vi "KickValueTest.vi"(8 "error in (no error)":errorcluster, 9 "grSIM replacement":T6, 10 "KickValueTest":T3={"ForceValue"={"delta_kick"=0.0, "kick_min"=1.0, "kick_max"=0.0}, "BallValue"={"delta_ball"=0.0, "v_min_ball"=1.0, "v_max_ball"=0.0}, "Samples"=0.0, "Start"=FALSE, "id"=0, "RobotStopKick"=FALSE}, 11 "Game in":refnum<class "Game.lvclass">) -> (0 "error out":errorcluster, 1 "KickValueState":T1 {"Progress" scale=0.0..100.0}, 2 "grSIM replacement out":T6, 3 "Game out":refnum<class "Game.lvclass">, 4 "replaceBall":bool, 5 "TestTeam":refnum<class "Ally.lvclass">, 6 "KickValue":dbl[][](array[numeric]), 7 "replaceRobots":bool)   [LabVIEW 2021, in "Game.lvclass"]
uses:
  Game.lvclass
  Controls/grSimReplacement.ctl
  Communication_class/Paths/grSim Packet Command UDP Test Folder/grSim/grSim RobotReplacement.ctl
  Communication_class/Paths/grSim Packet Command UDP Test Folder/grSim/grSim_BallReplacement.ctl
  Ally_class/Ally.lvclass
  D:/RoboIme/horie/SSL_AI/Team_class/Team.lvclass
  KickValuetest.ctl
  KickValue.ctl
  BallValue.ctl
  Kickvaluestate.ctl
  KickForceTest/Controls/KickForceEnum.ctl
  Game.lvclass/Game.ctl
  Team_class/Team.lvclass/Team.ctl
  Ball_class/Ball.lvclass/Ball.ctl
  Object_class/Object.lvclass/Object.ctl
  Robot_class/Robot.lvclass/Robot.ctl
  Events_class/Events.lvclass/Events.ctl
  RobotFeedback/RobotFeedback.lvclass/RobotFeedback.ctl
  <vilib>/Analysis/_algsub.llb/Real Vector Norm.vi
  Object_class/Read position(x,y).vi
  Events_class/Read kick.vi
  RobotFeedback/Read dribblerContactToBall.vi
  Robot_class/Write kick_x.vi
  Robot_class/Write v_tang.vi
  Robot_class/Write dribble.vi
  Read TestTeam.vi
  Read Utilities.lvclass.vi
  Read AllyRef.vi
  Read BallRef.vi
  Read FieldRef.vi
  Read EventsRef.vi
  Read RobotsFeedback.vi
  Ball_class/Read v_x.vi
  Ball_class/Read v_y.vi
  Object_class/Read x.vi
  Object_class/Read y.vi
  Team_class/Read RobotRef.vi
  Team_class/Write RobotRef.vi
  Ball_class/Ball.lvclass
  D:/RoboIme/horie/SSL_AI/Object_class/Object.lvclass
  Robot_class/Robot.lvclass
  Utilities_class/Utilities.lvclass
  Field_class/Field.lvclass
  Events_class/Events.lvclass
  RobotFeedback/RobotFeedback.lvclass
  <vilib>/Analysis/NI_AALPro.lvlib
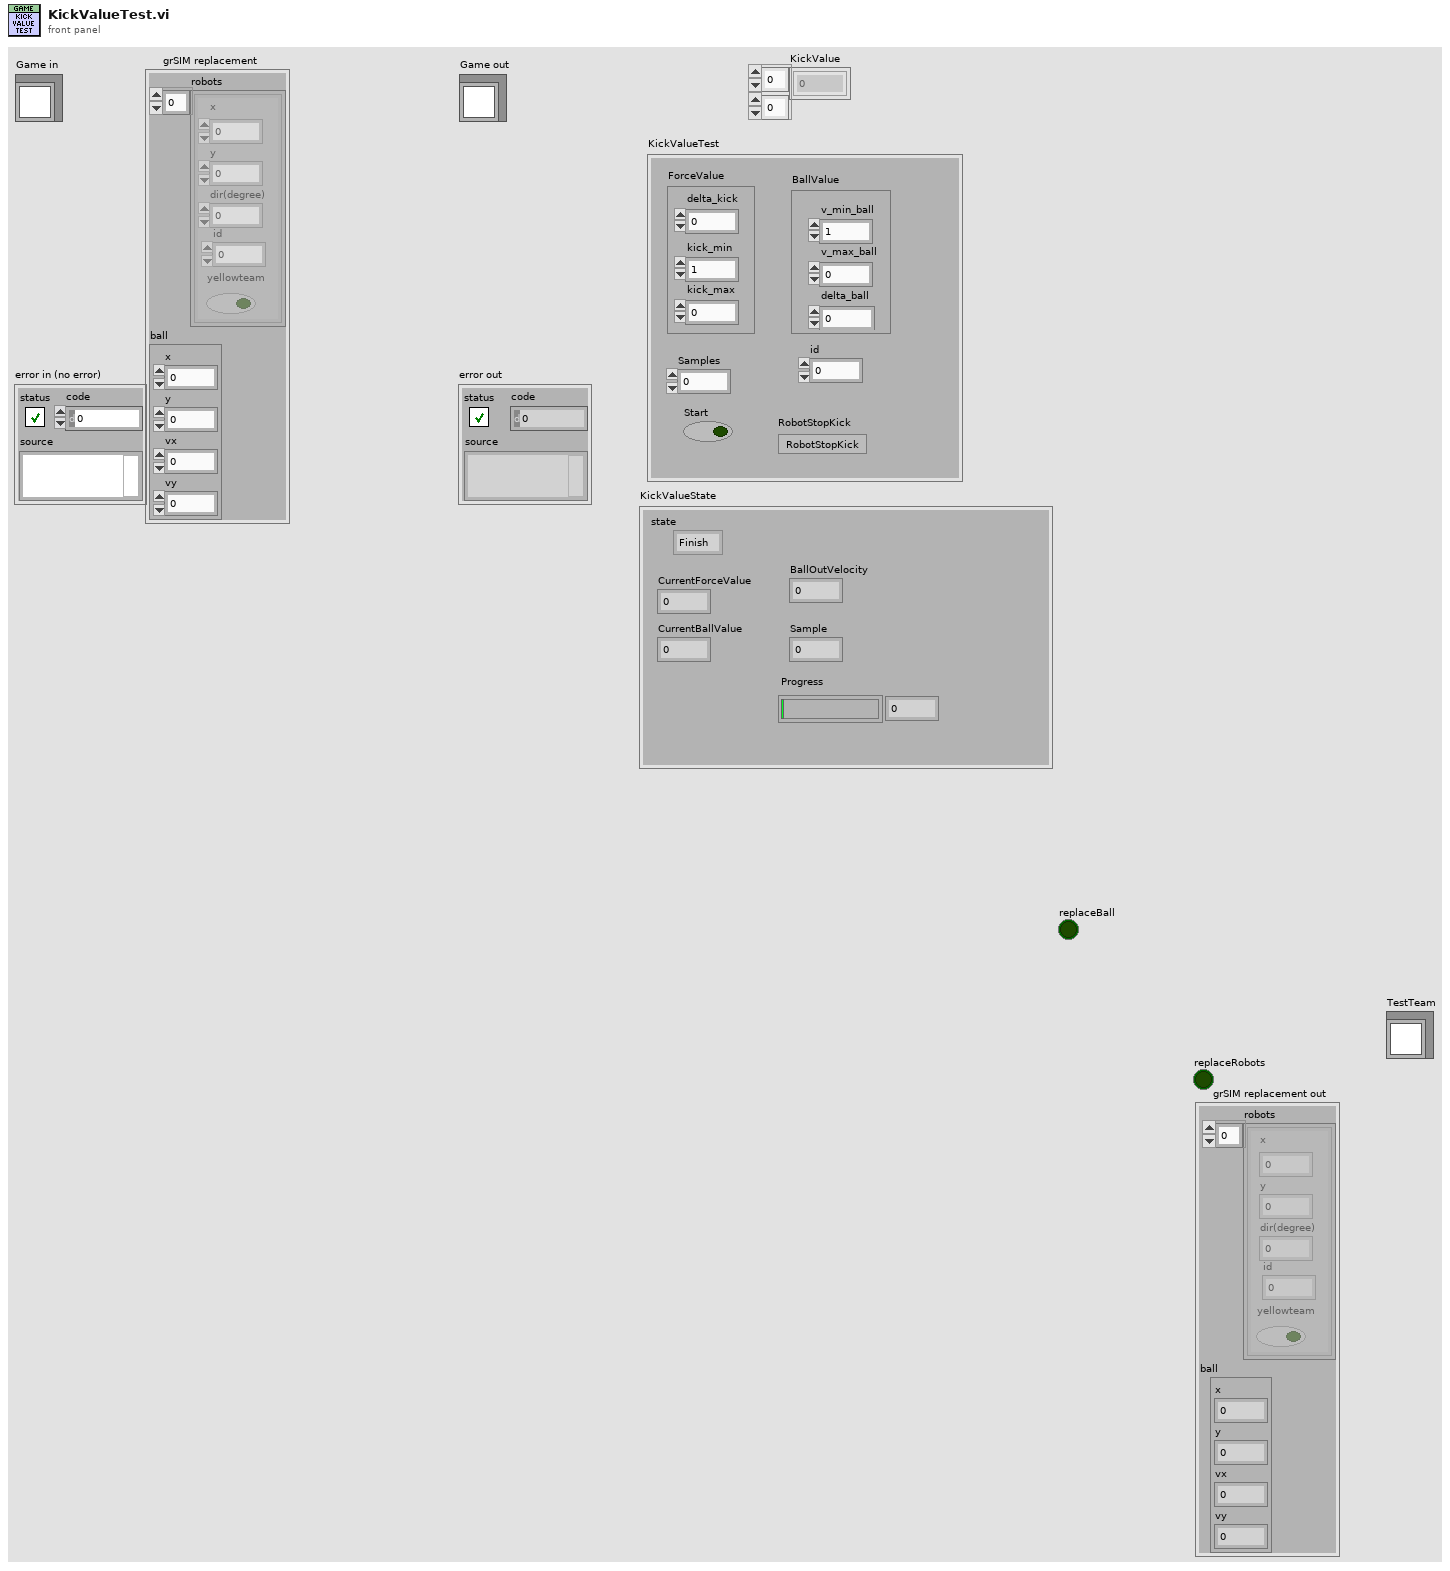
[diagram p1: front panel]
types:
  T1 = typedef "Game.lvclass/Kickvaluestate.ctl" = cluster{"state":T2, "CurrentForceValue":dbl, "CurrentBallValue":dbl, "BallOutVelocity":dbl, "Sample":dbl, "Progress":dbl}
  T2 = typedef "Game.lvclass/KickForceEnum.ctl" = enum16{"Finish", "Velball", "GoToNextKickForce", "WaitBall", "KickBall", "ReplaceBall"}
  T3 = typedef "KickValuetest.ctl" = cluster{"ForceValue":T4, "BallValue":T5, "Samples":dbl, "Start":bool, "id":i32, "RobotStopKick":bool}
  T4 = typedef "Game.lvclass/KickValue.ctl" = cluster{"delta_kick":dbl, "kick_min":dbl, "kick_max":dbl}
  T5 = typedef "Game.lvclass/BallValue.ctl" = cluster{"delta_ball":dbl, "v_min_ball":dbl, "v_max_ball":dbl}
  T6 = typedef "grSimReplacement.ctl" = cluster{"robots":T7[], "ball":T8}
  T7 = typedef "grSim RobotReplacement.ctl" = cluster{"x":dbl, "y":dbl, "dir(degree)":dbl, "yellowteam":bool, "id":u32}
  T8 = typedef "grSim_BallReplacement.ctl" = cluster{"x":dbl, "y":dbl, "vx":dbl, "vy":dbl}
  T9 = typedef "Kickmeanvalues.ctl" = dbl[][]
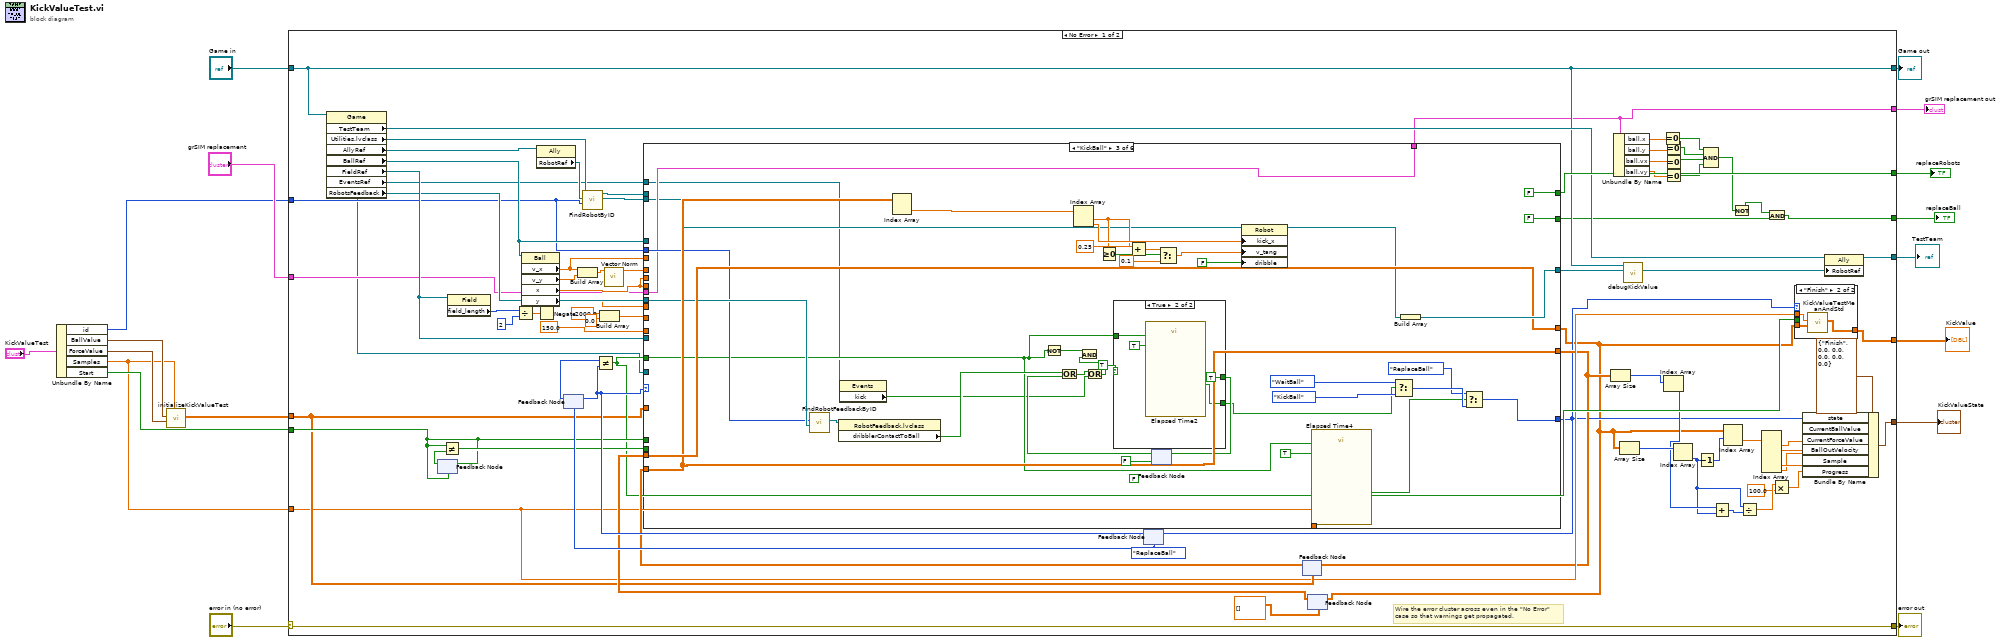
[diagram p0: block diagram]
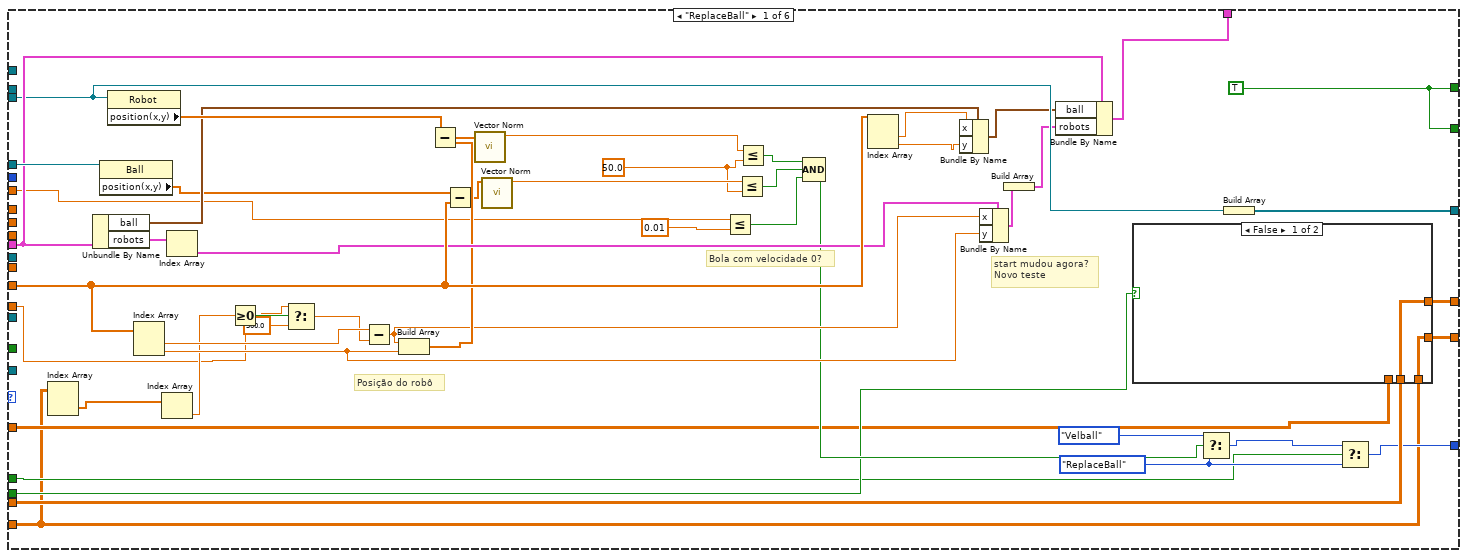
[diagram p3: hidden frame]
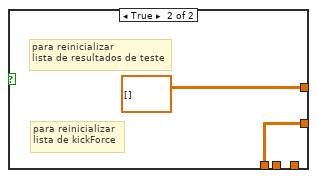
[diagram p4: hidden frame]
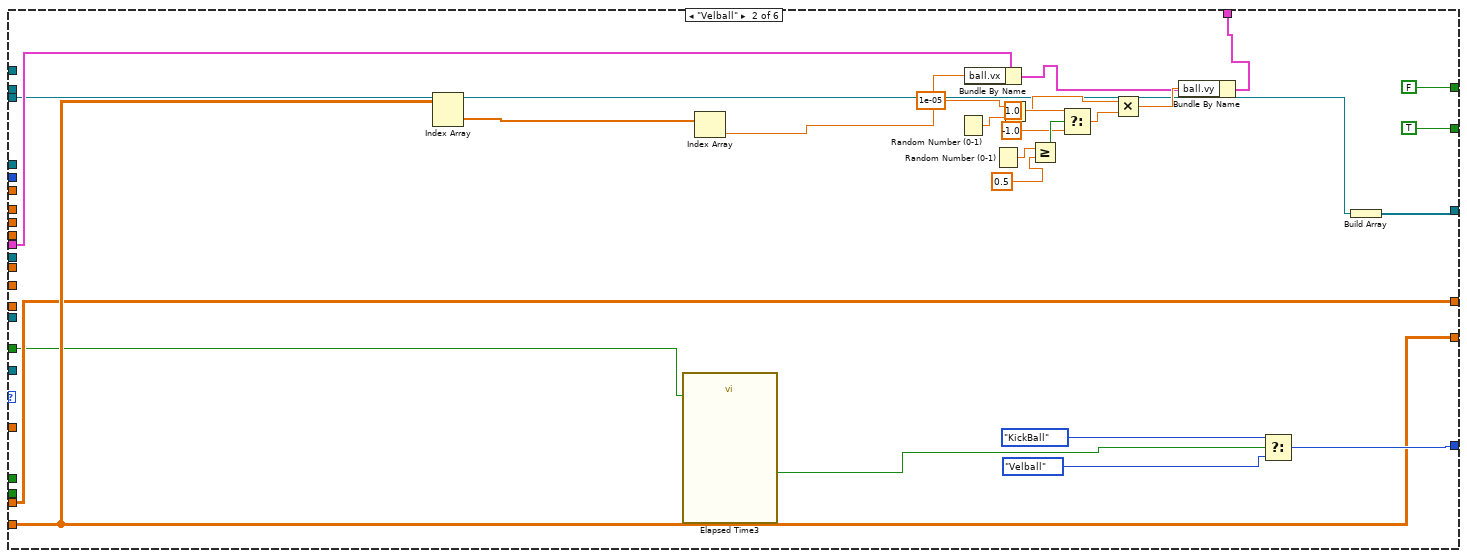
[diagram p5: hidden frame]
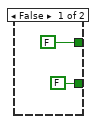
[diagram p6: hidden frame]
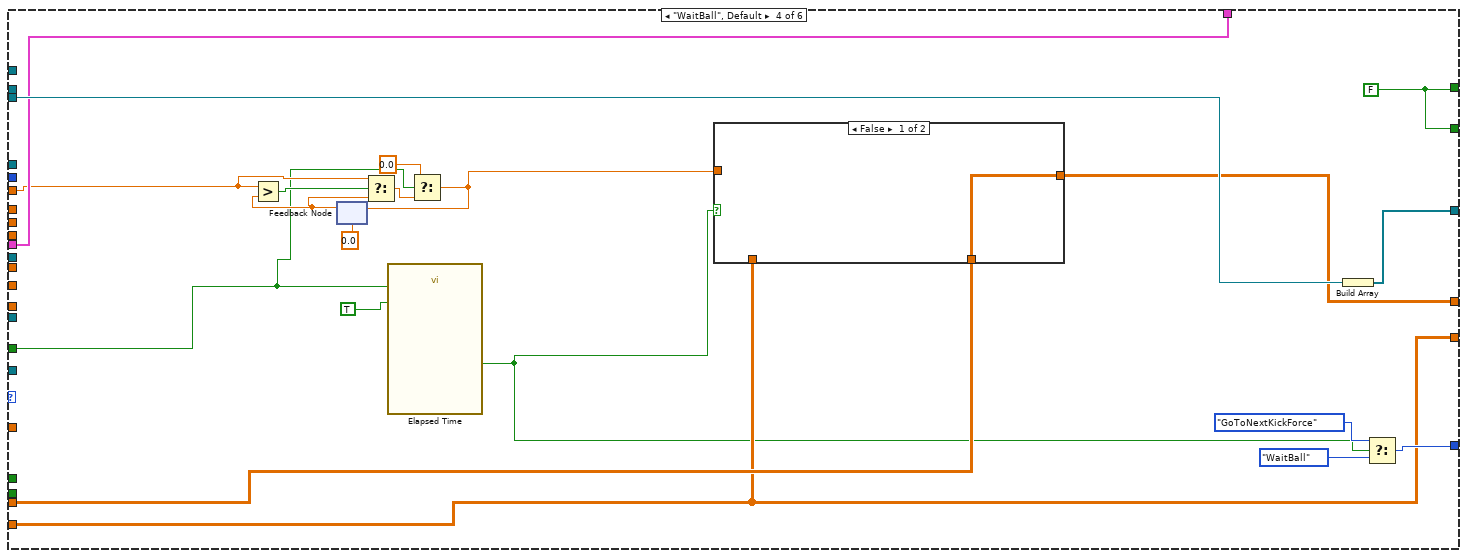
[diagram p7: hidden frame]
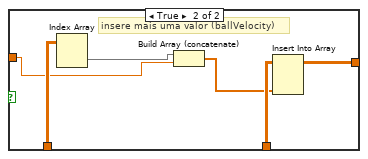
[diagram p8: hidden frame]
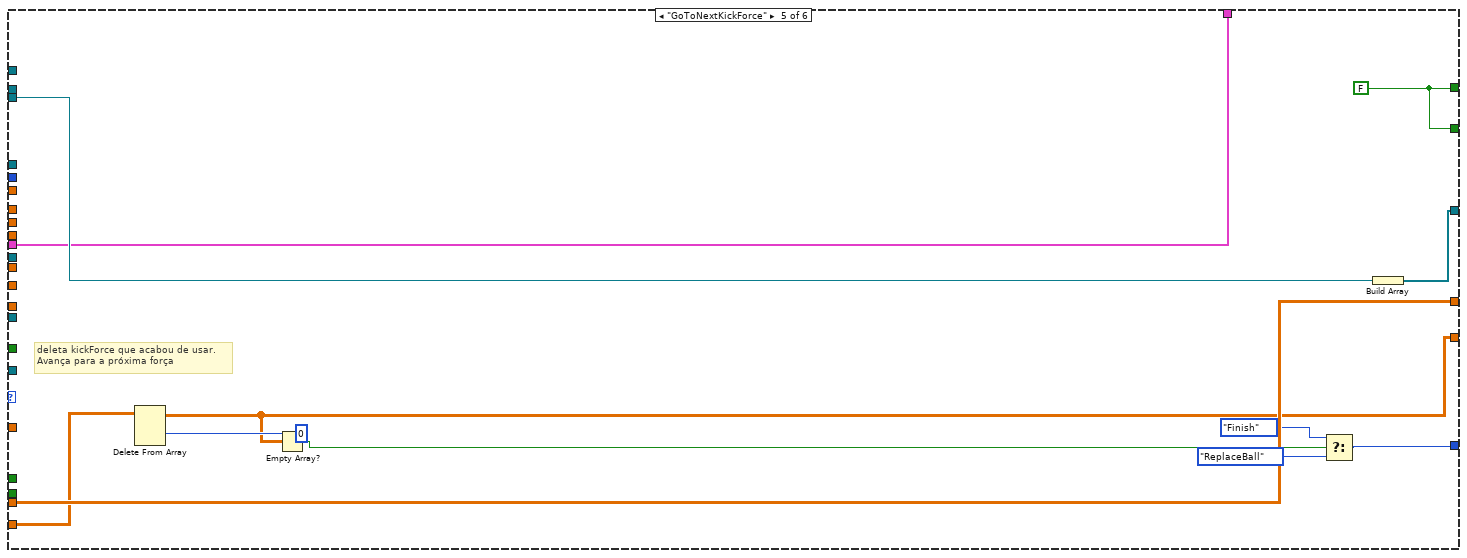
[diagram p9: hidden frame]
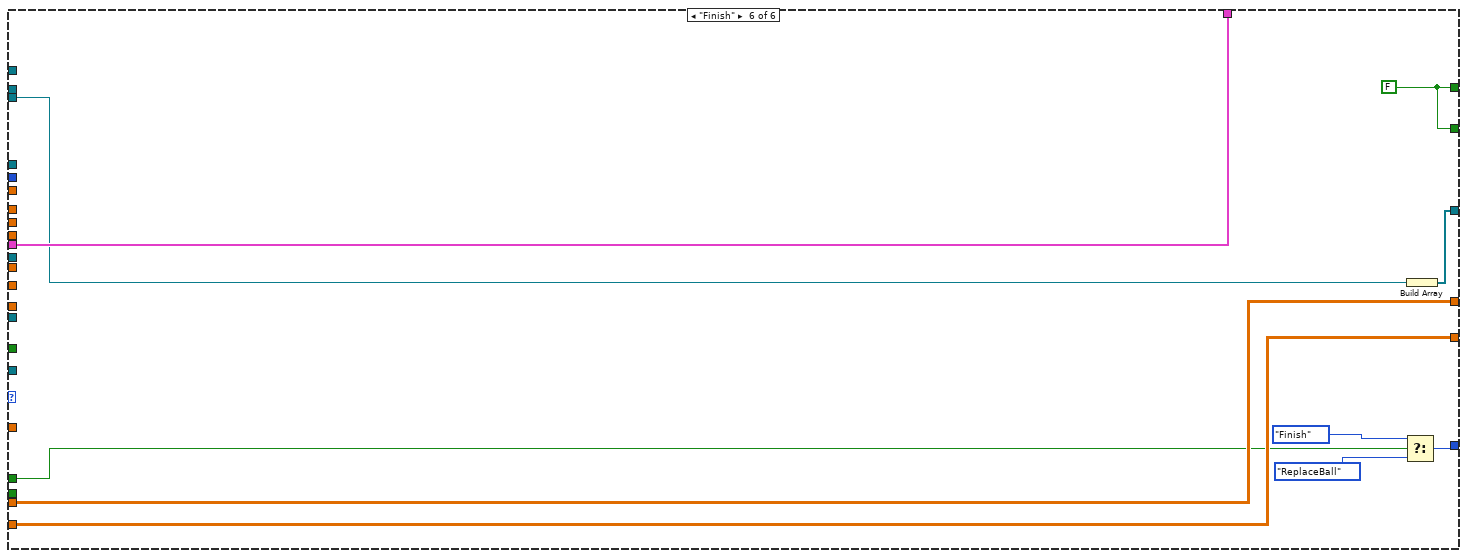
[diagram p10: hidden frame]
diagram:
  n1 = Unbundle By Name("KickValueTest") -> ("id"=w10:i32, "BallValue"=w11:T5, "ForceValue"=w12:T4, "Samples"=w7:dbl, "Start"=w9:bool)
  n2 = call "initializeKickValueTest.vi"("samples"=w7, "ForceValue"=w12, "BallValue"=w11) -> ("kickForceList"=w8:dbl[][])  [unwired: 6 in, 2 out]
  n3 = case shown="No Error" "error in (no error)" {
    selector: "error in (no error)" -> [w94 w272]
    tunnel: [w94 w272] -> w17
    tunnel: [w55 w271] -> w15
    tunnel: "Game in" -> [w55 w271]
    tunnel: w10 -> [w52 _]
    tunnel: w9 -> [w74 _]
    tunnel: "grSIM replacement" -> [w40 _]
    tunnel: w8 -> [w59 _]
    tunnel: w7 -> [w23 _]
    tunnel: [w70 _] -> w6
    tunnel: [w35 _] -> w5
    tunnel: [w69 _] -> w4
    tunnel: [w58 _] -> w3
    tunnel: [w67 _] -> w2
    tunnel: [w37 _] -> w1
    frame No Error {
      w77 = KickForceEnum."ReplaceBall" ("kickForceEnum")
      # "Wire the error cluster across even in the \"No Error\"\ncase so that warnings get propagated."
      n4 = property class="Game"(reference=w55) -> ("TestTeam"=w68:refnum<class "Ally.lvclass">, "Utilities.lvclass"=w91:refnum<class "Utilities.lvclass">, "AllyRef"=w93:refnum<class "Ally.lvclass">, "BallRef"=w86:refnum<class "Ball.lvclass">, "FieldRef"=w82:refnum<class "Field.lvclass">, "EventsRef"=w19:refnum<class "Events.lvclass">, "RobotsFeedback"=w53:refnum<class "RobotFeedback.lvclass">[])  [unwired: 1 in, 2 out]
      n5 = feedback #1(w74) -> (w76:bool)
      n6 = feedback-in #1(w74) -> ()
      n7 = Not Equal?(x=w74, y=w76) -> (x != y?=w75:bool)
      n8 = property class="Field"(reference=w82) -> ("field_length"=w85:i32)  [unwired: 1 in, 2 out]
      n9 = Divide(x=w85, y=2) -> (x/y=w83:dbl)
      n10 = property class="Ball"(reference=w86) -> ("v_x"=w54:dbl, "v_y"=w88:dbl, "x"=w42:dbl, "y"=w41:dbl)  [unwired: 1 in, 2 out]
      n11 = property class="Ally"(reference=w93) -> ("RobotRef"=w92:refnum<class "Robot.lvclass">[])  [unwired: 1 in, 2 out]
      n12 = Negate(x=w83) -> ()  [unwired: 1 out]
      n13 = feedback #2(w77) -> (w79:T2)
      n14 = Build Array(w54, w88) -> (w87:dbl[])
      n15 = call "FindRobotByID.vi"("id"=w52, "RobotRef"=w92, "Utilities in"=w91) -> ("Robot"=w89:refnum<class "Robot.lvclass">, "Utilities out"=w90:refnum<class "Utilities.lvclass">)  [unwired: 5 in, 2 out]
      n16 = Build Array(-2000.0 ("element"), 0.0 ("element")) -> (w81:dbl[])
      n17 = call-poly <vilib>:"Vector Norm.vi"("Input Vector"=w87) -> ("norm"=w36:dbl)  [unwired: 9 in, 1 out]
      n18 = feedback #3(w77) -> (w78:T2)
      n19 = feedback-in #2(w78) -> ()
      n20 = Not Equal?(x=w79, y=w78) -> (x != y?=w60:bool)
      n21 = feedback #4(w59) -> (w73:dbl[][])
      n22 = feedback #5(dbl[][] []) -> (w71:dbl[][])
      n23 = case shown="\"KickBall\"" w78 {
        tunnel: [w141 w173 w215 w240 w257 w266] -> w57
        tunnel: [w110 FALSE ("replaceRobots") FALSE ("replaceRobots") w232 w249 w261] -> w70
        tunnel: w89 -> [w142 w157 w188 w241 w256 w267]
        tunnel: w86 -> [w146 _ _ _ _ _]
        tunnel: w40 -> [w145 w170 w189 w235 w255 w270]
        tunnel: [w144 w156 w189 w235 w255 w270] -> w35
        tunnel: w81 -> [w143 _ _ _ _ _]
        tunnel: 150.0 ("y") -> [w99 _ _ _ _ _]
        tunnel: [w106 w174 w185 w237 w251 w264] -> w21
        tunnel: w54 -> [w115 _ _ w228 _ _]
        tunnel: w71 -> [w116 w153 w213 w239 w260 w269]
        tunnel: [w140 w153 w213 w238 w260 w269] -> w20
        tunnel: w73 -> [w104 w169 w211 w236 w259 w268]
        tunnel: w82 -> [_ _ _ _ _ _]
        tunnel: [w118 w169 w211 w236 w250 w268] -> w22
        tunnel: w60 -> [_ w151 w182 w225 _ _]
        tunnel: w74 -> [w105 _ _ _ _ w265]
        tunnel: w59 -> [w111 _ _ _ _ _]
        tunnel: w90 -> [_ _ _ _ _ _]
        tunnel: w75 -> [w117 _ _ _ _ _]
        tunnel: w23 -> [_ _ _ _ _ _]
        tunnel: [w110 TRUE ("replaceRobots") FALSE ("replaceRobots") w232 w249 w261] -> w39
        tunnel: w19 -> [_ _ _ _ _ _]
        tunnel: w53 -> [_ _ w199 _ _ _]
        tunnel: w52 -> [_ _ w198 _ _ _]
        tunnel: w42 -> [_ _ _ _ _ _]
        tunnel: w42 -> [_ _ _ _ _ _]
        tunnel: w41 -> [_ _ _ _ _ _]
        tunnel: w36 -> [_ _ _ _ _ _]
        tunnel: w19 -> [_ _ w181 _ _ _]
        frame "ReplaceBall" {
          w107 = KickForceEnum."ReplaceBall" ("kickForceEnum")
          w120 = 50.0 ("y")
          w110 = TRUE ("replaceRobots")
          # "Bola com velocidade 0?"
          # "start mudou agora?\nNovo teste"
          # "Posição do robô"
          n24 = Index Array(array=w104) -> (element=w103:dbl[])  [unwired: 2 in]
          n25 = Unbundle By Name(w145) -> ("ball"=w135:T8, "robots"=w139:T7[])
          n26 = property class="Ball"(reference=w146) -> ("position(x,y)"=w123:dbl[])  [unwired: 1 in, 2 out]
          n27 = property class="Robot"(reference=w142) -> ("position(x,y)"=w138:dbl[])  [unwired: 1 in, 2 out]
          n28 = Index Array(array=w143) -> (element #1=w129:dbl, element #2=w126:dbl)  [unwired: 2 in]
          n29 = Index Array(array=w103) -> (element=w100:dbl)  [unwired: 1 in]
          n30 = Index Array(array=w139) -> (element=w133:T7)  [unwired: 1 in]
          n31 = Greater Or Equal To 0?(x=w100) -> (x >= 0?=w102:bool)
          n32 = Select(t=w99, s=w102, f=300.0) -> (s? t:f=w101:dbl)
          n33 = Subtract(x=w129, y=w101) -> (x-y=w127:dbl)
          n34 = Build Array(w127, w126) -> (w128:dbl[])
          n35 = Subtract(x=w138, y=w128) -> (x-y=w137:dbl[])
          n36 = Subtract(x=w123, y=w143) -> (x-y=w122:dbl[])
          n37 = call-poly <vilib>:"Vector Norm.vi"("Input Vector"=w137) -> ("norm"=w136:dbl)  [unwired: 9 in, 1 out]
          n38 = call-poly <vilib>:"Vector Norm.vi"("Input Vector"=w122) -> ("norm"=w121:dbl)  [unwired: 9 in, 1 out]
          n39 = Less Or Equal?(x=w115, y=0.01) -> (x <= y?=w113:bool)
          n40 = Less Or Equal?(x=w121, y=w120) -> (x <= y?=w119:bool)
          n41 = Less Or Equal?(x=w136, y=w120) -> (x <= y?=w125:bool)
          n42 = Compound Arithmetic op=AND(w125, w119, w113) -> (w124:bool)
          n43 = Index Array(array=w143) -> (element #1=w132:dbl, element #2=w109:dbl)  [unwired: 2 in]
          n44 = Bundle By Name(cluster=w135, "x"=w132, "y"=w109) -> (w134:T8)
          n45 = Bundle By Name(cluster=w133, "x"=w127, "y"=w126) -> (w131:T7)
          n46 = Build Array(w131) -> (w130:T7[])
          n47 = Bundle By Name(cluster=w145, "ball"=w134, "robots"=w130) -> (w144:T6)
          n48 = case shown="False" w117 {
            tunnel: [w148 dbl[][] []] -> w140
            tunnel: [w147 w149] -> w118
            tunnel: w111 -> [_ w149]
            tunnel: w116 -> [w148 _]
            tunnel: w104 -> [w147 _]
            frame False {
            }
            frame True {
              # "para reinicializar\nlista de resultados de teste"
              # "para reinicializar\nlista de kickForce"
            }
          }
          n49 = Select(t=KickForceEnum."Velball" ("kickForceEnum"), s=w124, f=w107) -> (s? t:f=w108:T2)
          n50 = Build Array(w142) -> (w141:refnum<class "Robot.lvclass">[])
          n51 = Select(t=w108, s=w105, f=w107) -> (s? t:f=w106:T2)
        }
        frame "Velball" {
          n52 = Index Array(array=w169) -> (element=w171:dbl[])  [unwired: 2 in]
          n53 = call "Elapsed Time3"("Reset"=w151) -> ("Time has Elapsed"=w152:bool)  [unwired: 11 in, 7 out]
          n54 = Index Array(array=w171) -> (element=w154:dbl)  [unwired: 1 in]
          n55 = Random Number (0-1)() -> (number: 0 to 1=w166:dbl)
          n56 = Bundle By Name(cluster=w170, "ball.vx"=w154) -> (w158:T6)
          n57 = Random Number (0-1)() -> (number: 0 to 1=w165:dbl)
          n58 = Multiply(x=1e-05 ("ball.vy"), y=w166) -> (x*y=w160:dbl)
          n59 = Greater Or Equal?(x=w165, y=0.5) -> (x >= y?=w164:bool)
          n60 = Select(t=1.0, s=w164, f=-1.0) -> (s? t:f=w161:dbl)
          n61 = Multiply(x=w160, y=w161) -> (x*y=w159:dbl)
          n62 = Bundle By Name(cluster=w158, "ball.vy"=w159) -> (w156:T6)
          n63 = Select(t=KickForceEnum."KickBall" ("kickForceEnum"), s=w152, f=KickForceEnum."Velball" ("kickForceEnum")) -> (s? t:f=w174:T2)
          n64 = Build Array(w157) -> (w173:refnum<class "Robot.lvclass">[])
        }
        frame "KickBall" {
          (unwired) FALSE ("Time has Elapsed")
          n65 = call "FindRobotFeedbackByID.vi"("RobotsFeedback"=w199, "id"=w198) -> ("RobotFeedback.lvclass"=w197:refnum<class "RobotFeedback.lvclass">)  [unwired: 6 in, 3 out]
          n66 = property class="RobotFeedback.lvclass"(reference=w197) -> ("dribblerContactToBall"=w196:bool)  [unwired: 1 in, 2 out]
          n67 = property class="Events"(reference=w181) -> ("kick"=w178:bool)  [unwired: 1 in, 2 out]
          n68 = Index Array(array=w211) -> (element=w212:dbl[])  [unwired: 2 in]
          n69 = Not(x=w182) -> (.not. x?=w191:bool)
          n70 = Index Array(array=w212) -> (element #1=w200:dbl, element #2=w210:dbl)  [unwired: 2 in]
          n71 = Greater Or Equal To 0?(x=w200) -> (x >= 0?=w209:bool)
          n72 = case shown="True" TRUE {
            tunnel: [FALSE ("Time has Elapsed") w221] -> w192
            tunnel: [FALSE ("Time has Elapsed") TRUE ("Time has Elapsed")] -> w194
            tunnel: w182 -> [_ w218]
            frame False {
            }
            frame True {
              n73 = call "Elapsed Time2"("Reset"=w218, "Auto Reset"=TRUE) -> ("Time has Elapsed"=w221:bool)  [unwired: 10 in, 7 out]
            }
          }
          n74 = Add(x=w200, y=0.25) -> (x+y=w208:dbl)
          n75 = feedback-in #6(w194) -> ()
          n76 = feedback #6(FALSE ("Time has Elapsed")) -> (w195:bool)
          n77 = Or(x=w196, y=w195) -> (x .or. y?=w179:bool)
          n78 = Or(x=w179, y=w178) -> (x .or. y?=w180:bool)
          n79 = And(x=w191, y=w180) -> ()  [unwired: 1 out]
          n80 = Select(t=w208, s=w209, f=0.1) -> (s? t:f=w205:dbl)
          n81 = property class="Robot"(reference=w188, "kick_x"=w210, "v_tang"=w205, "dribble"=FALSE) -> (reference out=w204:refnum<class "Robot.lvclass">)  [unwired: 1 in, 1 out]
          n82 = call "Elapsed Time4"("Reset"=w182, "Auto Reset"=TRUE) -> ("Time has Elapsed"=w184:bool)  [unwired: 10 in, 7 out]
          n83 = Select(t=KickForceEnum."WaitBall" ("kickForceEnum"), s=w192, f=KickForceEnum."KickBall" ("kickForceEnum")) -> (s? t:f=w187:T2)
          n84 = Build Array(w204) -> (w215:refnum<class "Robot.lvclass">[])
          n85 = Select(t=KickForceEnum."ReplaceBall", s=w184, f=w187) -> (s? t:f=w185:T2)
        }
        frame "WaitBall", Default {
          w232 = FALSE ("replaceRobots")
          n86 = feedback #7(0.0 ("v_x")) -> (w229:dbl)
          n87 = Greater?(x=w228, y=w229) -> (0:w226:bool)
          n88 = Select(t=w228, s=w226, f=w229) -> (s? t:f=w224:dbl)
          n89 = call "Elapsed Time"("Reset"=w225, "Auto Reset"=TRUE) -> ("Time has Elapsed"=w231:bool)  [unwired: 10 in, 7 out]
          n90 = Select(t=0.0, s=w225, f=w224) -> (s? t:f=w222:dbl)
          n91 = feedback-in #7(w222) -> ()
          n92 = case shown="False" w231 {
            tunnel: w239 -> [w242 w248]
            tunnel: [w242 w247] -> w238
            tunnel: w236 -> [_ w246]
            tunnel: w222 -> [_ w243]
            frame False {
            }
            frame True {
              # "insere mais uma valor (ballVelocity)"
              n93 = Index Array(array=w246) -> (element=w244:dbl[])  [unwired: 2 in]
              n94 = Build Array (concatenate)(w244, w243) -> (w245:dbl[])
              n95 = Insert Into Array(array=w248, new element=w245) -> (w247:dbl[][])  [unwired: 2 in]
            }
          }
          n96 = Build Array(w241) -> (w240:refnum<class "Robot.lvclass">[])
          n97 = Select(t=KickForceEnum."GoToNextKickForce" ("kickForceEnum"), s=w231, f=KickForceEnum."WaitBall" ("kickForceEnum")) -> (s? t:f=w237:T2)
        }
        frame "GoToNextKickForce" {
          w249 = FALSE ("replaceRobots")
          # "deleta kickForce que acabou de usar.\nAvança para a próxima força"
          n98 = Delete From Array(array=w259, index (row)=0 ("index")) -> (array with subset deleted=w250:dbl[][])  [unwired: 2 in, 1 out]
          n99 = Empty Array?(array=w250) -> (empty?=w254:bool)
          n100 = Select(t=KickForceEnum."Finish" ("f"), s=w254, f=KickForceEnum."ReplaceBall") -> (s? t:f=w251:T2)
          n101 = Build Array(w256) -> (w257:refnum<class "Robot.lvclass">[])
        }
        frame "Finish" {
          w261 = FALSE ("replaceRobots")
          n102 = Select(t=KickForceEnum."Finish" ("kickForceEnum"), s=w265, f=KickForceEnum."ReplaceBall" ("kickForceEnum")) -> (s? t:f=w264:T2)
          n103 = Build Array(w267) -> (w266:refnum<class "Robot.lvclass">[])
        }
      }
      n104 = feedback-in #3(w21) -> ()
      n105 = feedback-in #4(w22) -> ()
      n106 = feedback-in #5(w20) -> ()
      n107 = Array Size(array=w22) -> (size(s)=w49:i32[])
      n108 = Unbundle By Name(w35) -> ("ball.x"=w34:dbl, "ball.y"=w33:dbl, "ball.vx"=w32:dbl, "ball.vy"=w31:dbl)
      n109 = Array Size(array=w20) -> (size(s)=w51:i32[])
      n110 = call "debugKickValue.vi"("RoboRefArray in"=w57, "Game in"=w55) -> ("RoboRefArray out"=w56:refnum<class "Robot.lvclass">[])  [unwired: 7 in, 2 out]
      n111 = Equal To 0?(x=w34) -> (x = 0?=w30:bool)
      n112 = Equal To 0?(x=w33) -> (x = 0?=w29:bool)
      n113 = Equal To 0?(x=w32) -> (x = 0?=w28:bool)
      n114 = Equal To 0?(x=w31) -> (x = 0?=w27:bool)
      n115 = Index Array(array=w49) -> (element=w47:i32)  [unwired: 1 in]
      n116 = Index Array(array=w51) -> (element=w43:i32)  [unwired: 1 in]
      n117 = Decrement(x=w43) -> (x-1=w50:i32)
      n118 = Compound Arithmetic op=AND(w30, w29, w28, w27) -> (w26:bool)
      n119 = Add(x=w47, y=w43) -> (x+y=w48:i32)
      n120 = Index Array(array=w20, index (row)=w50) -> (element=w65:dbl[])  [unwired: 1 in]
      n121 = Not(x=w26) -> (.not. x?=w38:bool)
      n122 = Divide(x=w43, y=w48) -> (x/y=w46:dbl)
      n123 = Index Array(array=w65) -> (element #1=w64:dbl, element #2=w63:dbl, element #5=w62:dbl, element #6=w61:dbl)  [unwired: 6 in, 2 out]
      n124 = And(x=w38, y=w39) -> (x .and. y?=w37:bool)
      n125 = Multiply(x=w46, y=100.0) -> (x*y=w45:dbl)
      n126 = case shown="\"Finish\"" w21 {
        tunnel: w60 -> [_ _]
        tunnel: w20 -> [_ w97]
        tunnel: [_ w96] -> w58
        tunnel: w23 -> [_ w95]
        frame Default {
        }
        frame "Finish" {
          n127 = call "KickValueTestMeanAndStd.vi"("ResultKickForce2DArray"=w97, "Sample"=w95) -> ("KickForceMean"=w96:T9)  [unwired: 8 in, 1 out]
        }
      }
      n128 = Bundle By Name(cluster=T1 {"state"=enum."Finish", "CurrentForceValue"=0.0, "CurrentBallValue"=0.0, "BallOutVelocity"=0.0, "Sample"=0.0, "Progress"=0.0} ("KickValueState"), "state"=w21, "CurrentBallValue"=w64, "CurrentForceValue"=w63, "BallOutVelocity"=w61, "Sample"=w62, "Progress"=w45) -> (w67:T1)
      n129 = property class="Ally"(reference=w68, "RobotRef"=w56) -> (reference out=w69:refnum<class "Ally.lvclass">)  [unwired: 1 in, 1 out]
    }
    frame Error {
    }
  }
  "error out" <- w17
  "Game out" <- w15
  "replaceRobots" <- w6
  "grSIM replacement out" <- w5
  "TestTeam" <- w4
  "replaceBall" <- w1
  "KickValue" <- w3
  "KickValueState" <- w2
